vi "Log.CreateTimeInfo.vi"() -> (2 "String":string, 3 "File Folder":path)   [LabVIEW 2015, in "Simple Sequence Tools - Shared.lvlib"]
uses:
  Simple Sequence Tools - Shared.lvlib
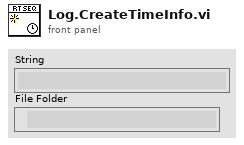
[diagram p1: front panel]
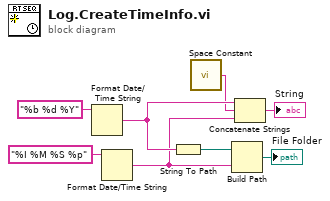
[diagram p0: block diagram]
diagram:
  n1 = Format Date/Time String(time format string (%c)="%b %d %Y") -> (date/time string=w4:string)  [unwired: 2 in]
  n2 = Format Date/Time String(time format string (%c)="%I %M %S %p") -> (date/time string=w3:string)  [unwired: 2 in]
  n3 = String To Path(string=w4) -> (path=w7:path)
  n4 = call <vilib>:"Space Constant.vi"() -> ("String"=w2:string)
  n5 = Build Path(base path=w7, name or relative path=w3) -> (appended path=→"File Folder":path)
  n6 = Concatenate Strings(w4, w2, w3) -> (→"String":string)
